vi "ER2007 Background DAQ Loop.vi"() -> ()   [LabVIEW 2013]
uses:
  <vilib>/Platform/TimedLoop/XDataNode/timing_clust.ctl
  <vilib>/Platform/TimedLoop/XDataNode/nitl_modes.ctl
  <vilib>/Platform/TimedLoop/XDataNode/wakeup.ctl
  <vilib>/DAQmx/read.llb/DAQmx Read (Analog 2D DBL NChan NSamp).vi
  <vilib>/Analysis/baseanly.llb/Mean (DBL).vi
  Controls/Global ER2007.vi
  <vilib>/DAQmx/create/channels.llb/DAQmx Create Channel (AI-Voltage-Basic).vi
  <vilib>/DAQmx/configure/timing.llb/DAQmx Timing (Sample Clock).vi
  <vilib>/DAQmx/miscellaneous.llb/DAQmx Fill In Error Info.vi
  <vilib>/platform/TimedLoop/XDataNode/XDataNode.xnode
  <vilib>/Analysis/NI_AALBase.lvlib
  <resource>/objmgr/daqmx.rc
  <vilib>/Platform/TimedLoop/XDataNode/XDNodeRunTimeDep.lvlib
panel:
  in  "T= Log Error":bool=TRUE
  in  "T=Notify":bool=TRUE
  in  "T=Notify":bool=TRUE
  in  "ThermocoupleType":u16(ring)=3 items=["B", "E", "J", "K", "R", "S", "T", "N"]
  out "Dev2 Err":bool
  out "Volts 2":dbl[](array[numeric]) format="%.4f"
  out "EUs 2":dbl[](array[numeric]) format="%.3f"
  out "NumCals 2":i32=28
  out "msec 3":u32=102
  in  "PhyChls 2":tag="Dev2/ai0:3, Dev2/ai5:11, Dev2/ai13:19, Dev2/ai21:27, Dev2/ai29:31"
  in  "MaxVolts 2":dbl=5.0 format="%0.2f"
  in  "MiinVolts 2":dbl=-5.0 format="%0.2f"
  in  "InputCfg 2":i32(ring)=10083 items=["default"=-1, "RSE"=10083, "NRSE"=10078, "Differential"=10106, "Pseudodifferential"=12529]
  in  "Rate 2":dbl=1000.0
  in  "SampleMode 2":i32(ring)=10178 items=["Finite Samples"=10178, "Continuous Samples"=10123, "Hardware Timed Single Point"=12522]
  in  "Samps/Chl 2":i32=100
  out "NumChls 3":i32=28
  out "ActRate 2":dbl format="%.2f"
  out "Sample 2":bool
  out "Galil Err":bool
  out "Dev1 Err":bool
  out "EUs 1":dbl[](array[numeric]) format="%.3f"
  out "Sample 1":bool
  out "Query":bool
  out "NumCtrls":i32
  in  "Controller #'s":u16[](array[numeric])=[1, 1, 1, 1, 1]
  out "msec 2":u32=102
  out "msec 1":u32=102
  out "ActRate":dbl format="%.2f"
  out "EUs 3":dbl[](array[numeric]) format="%.2f"
  in  "TC & CJ-1 Idxs":i32[][](array[numeric])=[[1, 5], [2, 6], [8, 15], [9, 16], [12, 19], [13, 20], [22, 29], [23, 30], [26, 33], [27, 34]]
  out "NumCals 3":i32=10
  out "NumCals 1":i32=7
  out "Late":bool
  out "Volts 1":dbl[](array[numeric]) format="%.4f"
  out "NumChls 3":i32=10
  out "NumChls 1":i32=7
  in  "Devs":T1(ring)=enum."All"
  in  "Period 3":dbl=60.0 caption="(secs)"
  out "ErrOut":errorcluster
  in  "Samps/Chl 1":i32=100
  in  "SampleMode 1":i32(ring)=10178 items=["Finite Samples"=10178, "Continuous Samples"=10123, "Hardware Timed Single Point"=12522]
  in  "Rate 1":dbl=1000.0
  in  "InputCfg 1":i32(ring)=10083 items=["default"=-1, "RSE"=10083, "NRSE"=10078, "Differential"=10106, "Pseudodifferential"=12529]
  in  "MiinVolts 1":dbl=-5.0 format="%0.2f"
  in  "MaxVolts 1":dbl=5.0 format="%0.2f"
  in  "SimOn":bool
  in  "Stop":bool
  in  "PhyChls 1":tag="Dev1/ai0:3, Dev1/ai8:10"
  in  "Init":bool
  # "Dev 1"
  # "Galil CDS-3310"
  # "Note: Max rate is about 8333 Hz (250 Khz / 30 chls)"
  # "Pvol1"
  # "Pdp2"
  # "Pvol2"
  # "Pdp3"
  # "Pdp4"
  # "Pdp5"
  # "Pvol5"
  # "Dev 2"
  # "Galil Assignments\n\nNet Chl  Chl Desc  Dev Out Idx  Both Dev Idx\n-------  --------  -----------  ------------\nNet 0.1   DelP1          0           35\nNet 0.2    Vol1          1           36\nNet 1.1   Delp2          2           37\nNet 1.2    Vol2          3           38\nNet 2.1   DelP3          4           39\nNet 2.2    Vol3          5           40\nNet 3.1   DelP4          6           41\nNet 3.2    Vol4          7           42\nNet 4.1   DelP5          8           43\nNet 4.2    Vol5          9           44"
  # "Old ER2006 Dev 1 Assignments\n\nA/D Chl  Chl Desc  Dev Out Idx  Both Dev Idx\n-------  --------  -----------  ------------\n    0      NOP1          0            0\n    1      TC1A          1            1\n    2      TC1B          2            2\n    3      NOP2          3            3\n    4      TC2A          4            4\n    5      TC2B          5            5\n    6      NOP3          6            6\n    7    <spare>         -            -\n    8       Pc1          7            7\n    9      CJ1A          8            8\n   10      CJ1B          9            9\n   11       Pc2         10           10\n   12      CJ2A         11           11\n   13      CJ2B         12           12\n   14       Pc3         13           13\n   15    <spare>         -            -\n   16      TC3A         14           14\n   17      TC3B         15           15\n   18      NOP4         16           16\n   19      TC4A         17           17\n   20      TC4B         18           18\n   21      NOP5         19           19\n   22      TC5A         20           20\n   23      TC5B         21           21\n   24      CJ3A         22           22\n   25      CJ3B         23           23\n   26       Pc4         24           24\n   27      CJ4A         25           25\n   28      CJ4B         26           26\n   29       Pc5         27           27\n   30      CJ5A         28           28\n   31      CJ5B         29           29"
  # "Dev 1 PCI-6220 Assignments\n\nA/D Chl  Chl Desc  Dev Out Idx  Both Dev Idx\n-------  --------  -----------  ------------\n    0      NOP1          0            0\n    1      TC1A          1            1\n    2      TC1B          2            2\n    3      Pc1B          3            3\n    4    <spare>         -            -\n    5    <spare>         -            -\n    6    <spare>         -            -\n    7    <spare>         -            -\n    8      Pc1A          4            4\n    9      CJ1A          5            5\n   10      CJ1B          6            6"
  # "Dev 2 PCI-6224 Assignments\n\nA/D Chl  Chl Desc  Dev Out Idx  Both Dev Idx\n-------  --------  -----------  ------------\n    0      NOP2          0            7\n    1      TC2A          1            8\n    2      TC2B          2            9\n    3      Pc2B          3           10\n    4    <spare>         -            -\n    5      Pc3A          4           11\n    6      TC3A          5           12\n    7      TC3B          6           13\n    8      Pc2A          7           14\n    9      CJ2A          8           15\n   10      CJ2B          9           16\n   11      NOP3         10           17\n   12    <spare>         -            -\n   13      Pc3B         11           18\n   14      CJ3A         12           19\n   15      CJ3B         13           20\n   16      NOP4         14           21\n   17      TC4A         15           22\n   18      TC4B         16           23\n   19      Pc4B         17           24\n   20    <spare>         -            -\n   21      Pc5A         18           25\n   22      TC5A         19           26\n   23      TC5B         20           27\n   24      Pc4A         21           28\n   25      CJ4A         22           29\n   26      CJ4B         23           30\n   27      NOP5         24           31\n   28    <spare>         -            -\n   29      Pc5B         25           32\n   30      CJ5A         26           33\n   31      CJ5B         27           34"
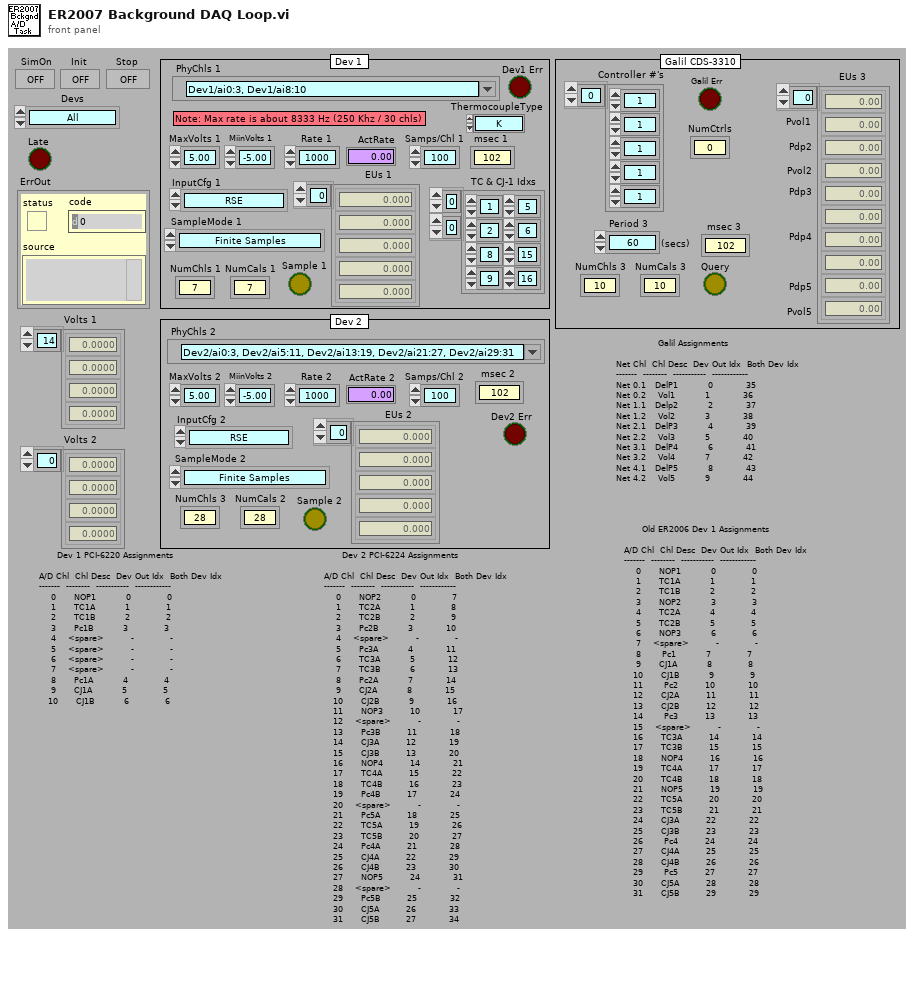
[diagram p1: front panel]
types:
  T1 = enum16{"Dev 1", "Dev 2", "Dev 1 & Dev 2", "Galil", "All"}
  T2 = typedef "XDNodeRunTimeDep.lvlib/timing_clust.ctl" = cluster{"Expected End [f-1]":u64, "Actual End [f-1]":u64, "Finished Late? [f-1]":bool, "Expected End [i-1]":u64, "Actual End [i-1]":u64, "Finished Late? [i-1]":bool, "Expected Start [i]":u64, "Actual Start [i]":u64, "Expected Start [f]":u64, "Actual Start [f]":u64, "Source Name":string, "Structure Name":string, "Period":i64, "Deadline":i64, "Offset":i64, "Start":i64, "Priority":i32, "Timeout":i32, "Mode":T3, "Wakeup Reason":T4, "Error":errorcluster, "Source Type":string, "Secondary Source Type":string, "Global End Time":u64, "Global Start Time":u64, "Frame Duration":u64, "Iteration Duration":u64, "Assigned CPU":i32, "I/O Scan Engine Mode":u32}
  T3 = typedef "XDNodeRunTimeDep.lvlib/nitl_modes.ctl" = enum32{"No Change", "Process missed periods, maintain original phase", "Discard missed periods, maintain original phase", "Process missed periods, ignore original phase", "Discard missed periods, ignore original phase"}
  T4 = typedef "XDNodeRunTimeDep.lvlib/wakeup.ctl" = enum32{"Normal", "Aborted", "Asynchronous wakeup", "Timing source error", "Timed loop error", "Timeout"}
  T5 = cluster{"PageTitle":string, "NumLines":i32, "ChlNum":string[], "ChlDesc":string[], "ChlUnits":string[], "ChlZero":sgl[], "ChlFactor":sgl[], "ChlConfig":u16[]}[]
  T6 = cluster{"PageTitle":string, "NumLines":i32, "ChlNum":string[], "ChlDesc":string[], "ChlUnits":string[], "ChlZero":sgl[], "ChlFactor":sgl[], "ChlConfig":u16[]}
  T7 = enum16{"Cell 1", "Cell 2", "Cell 3", "Cell 4", "Cell 5"}
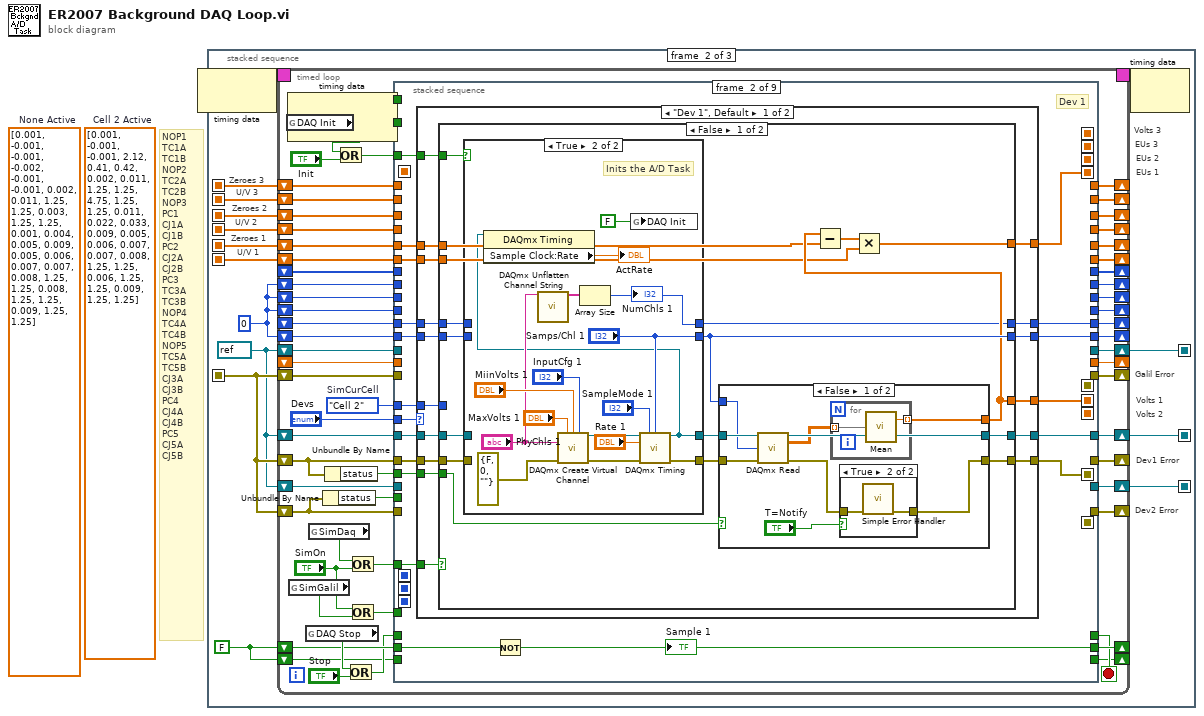
[diagram p0: block diagram]
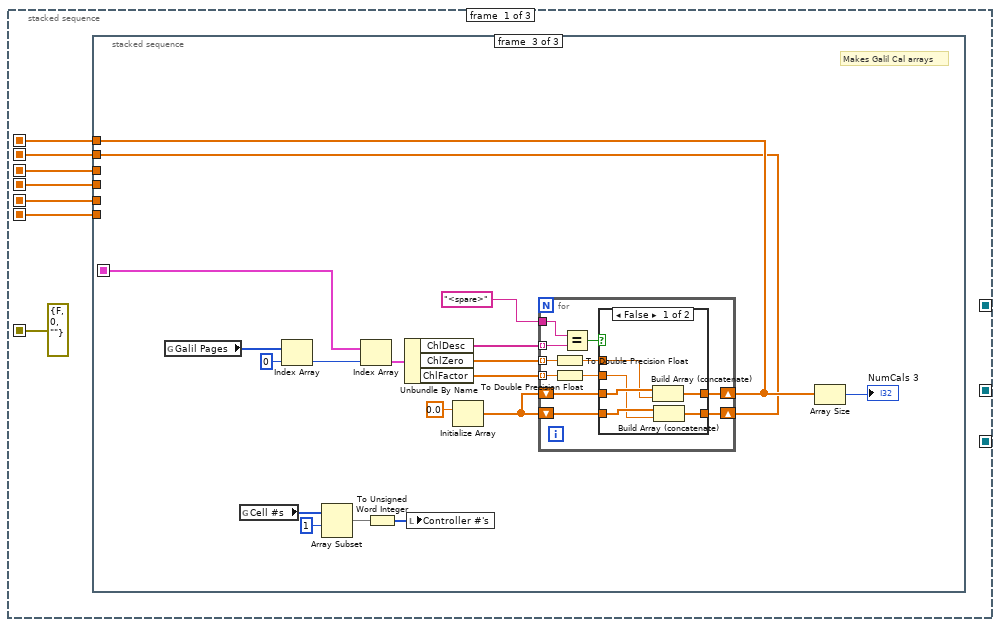
[diagram p2: hidden frame]
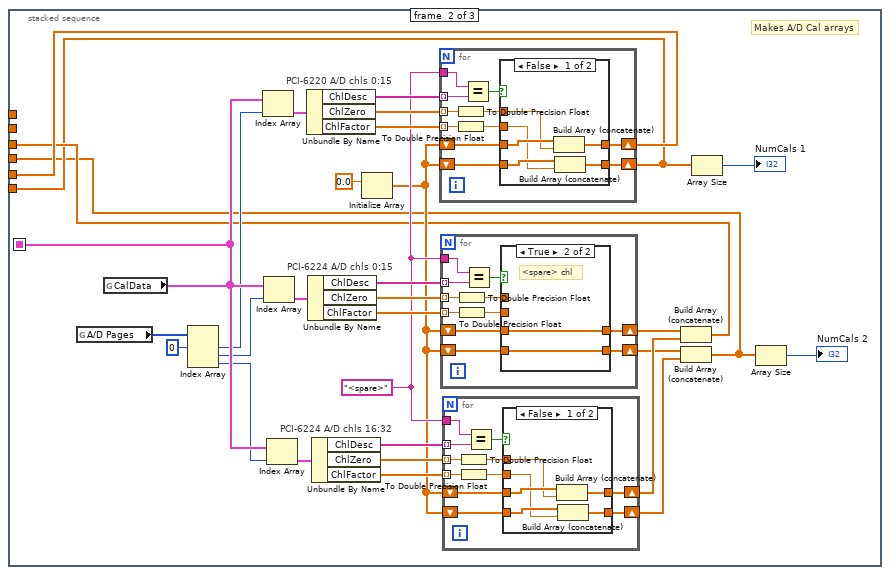
[diagram p4: hidden frame]
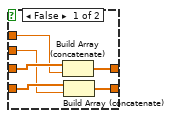
[diagram p7: hidden frame]
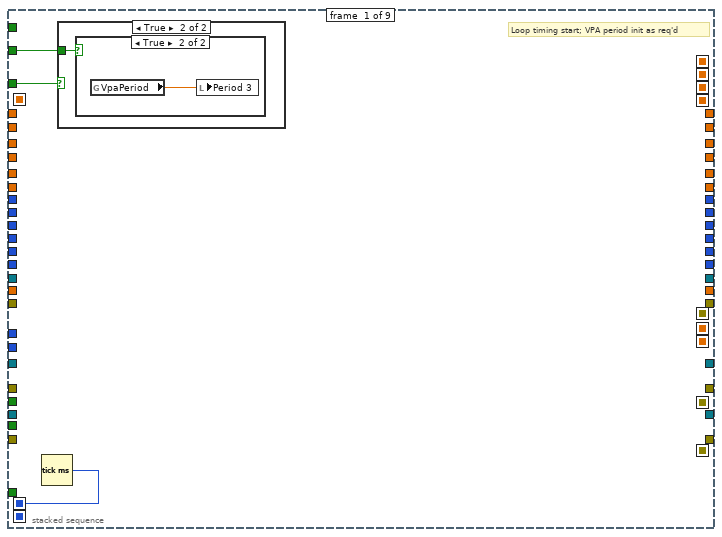
[diagram p9: hidden frame]
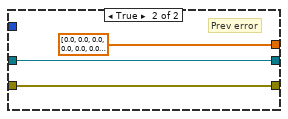
[diagram p13: hidden frame]
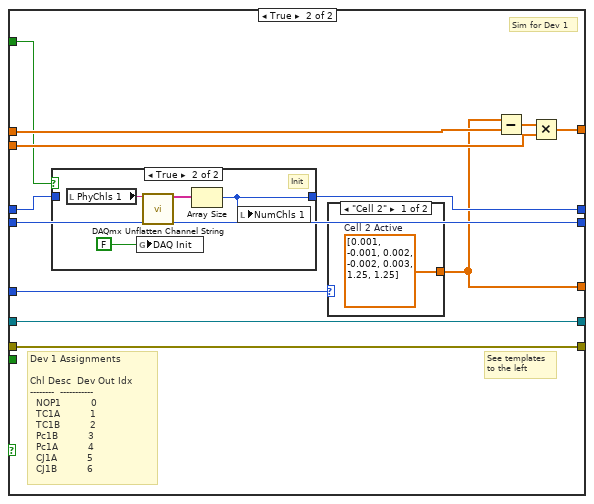
[diagram p15: hidden frame]
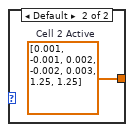
[diagram p16: hidden frame]
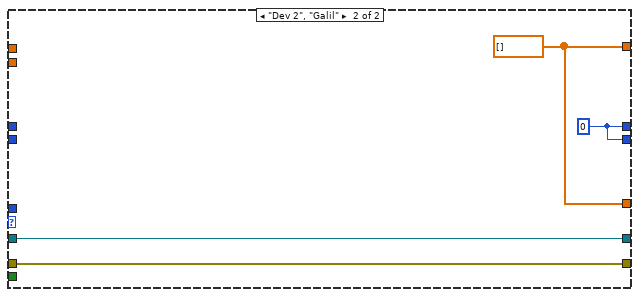
[diagram p18: hidden frame]
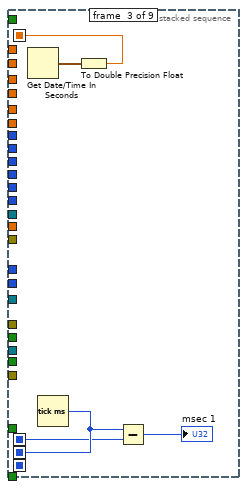
[diagram p19: hidden frame]
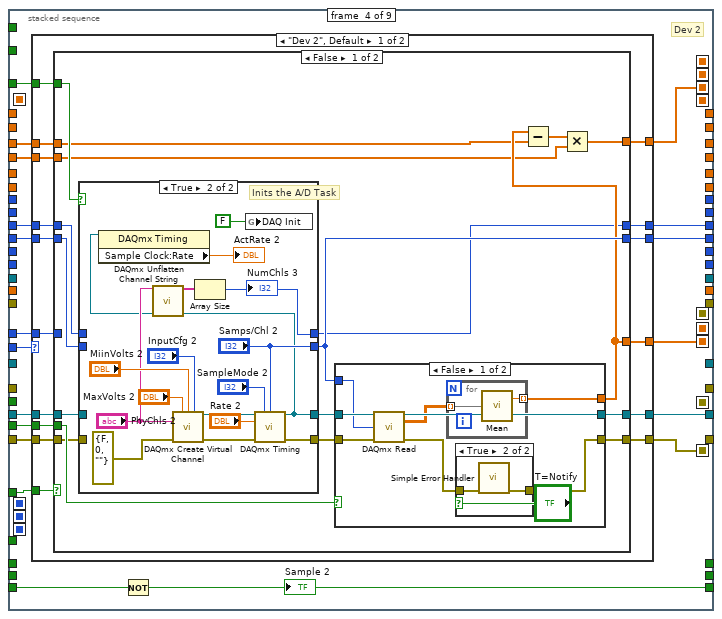
[diagram p20: hidden frame]
diagram:
  (unwired) dbl[] [0.001, -0.001, -0.001, 2.12, 0.41, 0.42, 0.002, 0.011, 1.25, 1.25, 4.75, 1.25, 1.25, 0.011, 0.022, 0.033, 0.009, 0.005, 0.006, 0.007, 0.007, 0.008, 1.25, 1.25, 0.006, 1.25, 1.25, 0.009, 1.25, 1.25]  # Cell 2 Active
  (unwired) dbl[] [0.001, -0.001, -0.001, -0.002, -0.001, -0.001, 0.002, 0.011, 1.25, 1.25, 0.003, 1.25, 1.25, 0.001, 0.004, 0.005, 0.009, 0.005, 0.006, 0.007, 0.007, 0.008, 1.25, 1.25, 0.008, 1.25, 1.25, 0.009, 1.25, 1.25]  # None Active
  # "NOP1\nTC1A\nTC1B\nNOP2\nTC2A\nTC2B\nNOP3\nPC1\nCJ1A\nCJ1B\nPC2\nCJ2A\nCJ2B\nPC3\nTC3A\nTC3B\nNOP4\nTC4A\nTC4B\nNOP5\nTC5A\nTC5B\nCJ3A\nCJ3B\nPC4\nCJ4A\nCJ4B\nPC5\nCJ5A\nCJ5B"
  n1 = stacked-sequence {
    seq-local: [w3 _ _] -> [_ w136 _]
    seq-local: [w7 _ _] -> [_ w135 _]
    seq-local: [_ w147 _] -> [_ _ w876]
    seq-local: [w5 _ _] -> [_ w140 _]
    seq-local: [w6 _ _] -> [_ w139 _]
    seq-local: [_ w146 _] -> [_ _ w875]
    seq-local: [errorcluster {"status"=FALSE, "code"=0, "source"=""} ("error out") _ _] -> [_ w145 _]
    seq-local: [w2 _ _] -> [_ w138 _]
    seq-local: [w1 _ _] -> [_ w137 _]
    seq-local: [_ w141 _] -> [_ _ w873]
    frame #0 {
      n2 = stacked-sequence {
        seq-local: [_ w19 _] -> [_ _ w100]
        tunnel: [_ w11 _] -> w3
        tunnel: [_ w9 _] -> w7
        tunnel: [_ _ w98] -> w6
        tunnel: [_ _ w99] -> w5
        tunnel: [_ w10 _] -> w2
        tunnel: [_ w8 _] -> w1
        frame #0 {
          # "Notes and such"
          # "ERROR HANDLING\n\nTwo types of errors are reported: A/D errors and Galil (VPA) errors.  Each of the two\ncode sections has its own error cluster which are are checked in frame #5.  Errors are\nreported to the Main Test Panel using two separate globals.\n\nA/D Errors\n----------\nA/D errors do not generally occur once the code is optimized and tested for the first time.\nErrors that do occur after initial testing are generally fatal and hardware related.  There\nis no attempt inside the A/D code to correct for errors or write errors to the error log file.\nA/D sample rates are about 1000 samples per seconds.\n\nOnce an A/D error occurs, the error is latched until the problem is fixed and either the\n\"Reset DAQ\" is pressed on the Main Test Panel or the program is restarted.\n\nGalil Errors\n------------\nGalil errors are much more common and arise from communication errors due to collisions or\ntimeouts, and to the user tinkering with the VPA hardware or software configuration.  Not only\nare genuine errors possible but the user can change the data collection method from auto-VPA\npolling to Manual on any of the five VPA's on-the-fly.  This Auto/Manual switch is handled\ninternally in the five VPA vi's.  VPA polling occurs at 60 second intervals.\n\nAfter an error occurs it is latched until a subsequent poll is successfully completed at which\ntime the error is automatically cleared.  During polling, the first VPA to report an error is\nlatched; polling of higher numbered VPA's continues as though there were no error in an effort\nto collect data from working VPA's.  Errors in higher numbered VPA's are not reported if an\nerror occurred in a lower numbered one.\n\nError Logging\n-------------\nLogging errors to an error file is done only for VPA errors.  Only the first error of\nsuccessive errors is logged; a \"no-error\" poll resets the error logging vi and re-arms it."
        }
        frame #1 {
          w18 = "<spare>" ("x")
          # "PCI-6220 A/D chls 0:15"
          # "Makes A/D Cal arrays"
          # "PCI-6224 A/D chls 16:32"
          # "PCI-6224 A/D chls 0:15"
          n3 = global read "Global ER2007.vi" "A/D Pages"() -> (w28:i32[])
          n4 = global read "Global ER2007.vi" "CalData"() -> (w19:T5)
          n5 = Index Array(array=w28, index #1=0 ("index")) -> (element #1=w14:i32, element #2=w15:i32, element #3=w16:i32)  [unwired: 2 in]
          n6 = Index Array(array=w19, index=w14) -> (element=w23:T6)
          n7 = Index Array(array=w19, index=w15) -> (element=w36:T6)
          n8 = Index Array(array=w19, index=w16) -> (element=w38:T6)
          n9 = Unbundle By Name(w23) -> ("ChlDesc"=w22:string[], "ChlZero"=w21:sgl[], "ChlFactor"=w20:sgl[])
          n10 = Unbundle By Name(w36) -> ("ChlDesc"=w35:string[], "ChlZero"=w34:sgl[], "ChlFactor"=w33:sgl[])
          n11 = Unbundle By Name(w38) -> ("ChlDesc"=w29:string[], "ChlZero"=w30:sgl[], "ChlFactor"=w31:sgl[])
          n12 = Initialize Array(0.0 ("element")) -> (w17:dbl[])  [unwired: 1 in]
          n13 = for {
            tunnel: w22 -> [w49] mode=indexing
            tunnel: w21 -> [w42] mode=indexing
            tunnel: w20 -> [w41] mode=indexing
            tunnel: w18 -> [w48]
            shift-right: [w45] -> w11
            shift-left: w17 -> [w46]
            shift-right: [w43] -> w9
            shift-left: w17 -> [w44]
            n14 = To Double Precision Float(number=w42) -> (double precision float=w40:dbl)
            n15 = To Double Precision Float(number=w41) -> (double precision float=w39:dbl)
            n16 = Equal?(x=w48, y=w49) -> (x = y?=w47:bool)
            n17 = case shown="False" w47 {
              tunnel: w46 -> [w55 w57]
              tunnel: [w53 w57] -> w45
              tunnel: w44 -> [w51 w56]
              tunnel: [w52 w56] -> w43
              tunnel: w40 -> [w54 _]
              tunnel: w39 -> [w50 _]
              frame False {
                n18 = Build Array (concatenate)(w55, w54) -> (w53:dbl[])
                n19 = Build Array (concatenate)(w51, w50) -> (w52:dbl[])
              }
              frame True {
                # "<spare> chl"
              }
            }
          }
          n20 = for {
            tunnel: w35 -> [w87] mode=indexing
            tunnel: w34 -> [w80] mode=indexing
            tunnel: w33 -> [w79] mode=indexing
            tunnel: w18 -> [w86]
            shift-right: [w83] -> w26
            shift-left: w17 -> [w84]
            shift-right: [w81] -> w24
            shift-left: w17 -> [w82]
            n21 = To Double Precision Float(number=w80) -> (double precision float=w78:dbl)
            n22 = To Double Precision Float(number=w79) -> (double precision float=w77:dbl)
            n23 = Equal?(x=w86, y=w87) -> (x = y?=w85:bool)
            n24 = case shown="True" w85 {
              tunnel: w84 -> [w93 w95]
              tunnel: [w91 w95] -> w83
              tunnel: w82 -> [w89 w94]
              tunnel: [w90 w94] -> w81
              tunnel: w78 -> [w92 _]
              tunnel: w77 -> [w88 _]
              frame False {
                n25 = Build Array (concatenate)(w93, w92) -> (w91:dbl[])
                n26 = Build Array (concatenate)(w89, w88) -> (w90:dbl[])
              }
              frame True {
                # "<spare> chl"
              }
            }
          }
          n27 = for {
            tunnel: w29 -> [w68] mode=indexing
            tunnel: w30 -> [w61] mode=indexing
            tunnel: w31 -> [w60] mode=indexing
            tunnel: w18 -> [w67]
            shift-right: [w64] -> w27
            shift-left: w17 -> [w65]
            shift-right: [w62] -> w25
            shift-left: w17 -> [w63]
            n28 = To Double Precision Float(number=w61) -> (double precision float=w59:dbl)
            n29 = To Double Precision Float(number=w60) -> (double precision float=w58:dbl)
            n30 = Equal?(x=w67, y=w68) -> (x = y?=w66:bool)
            n31 = case shown="False" w66 {
              tunnel: w65 -> [w74 w76]
              tunnel: [w72 w76] -> w64
              tunnel: w63 -> [w70 w75]
              tunnel: [w71 w75] -> w62
              tunnel: w59 -> [w73 _]
              tunnel: w58 -> [w69 _]
              frame False {
                n32 = Build Array (concatenate)(w74, w73) -> (w72:dbl[])
                n33 = Build Array (concatenate)(w70, w69) -> (w71:dbl[])
              }
              frame True {
                # "<spare> chl"
              }
            }
          }
          n34 = Build Array (concatenate)(w26, w27) -> (w10:dbl[])
          n35 = Build Array (concatenate)(w24, w25) -> (w8:dbl[])
          n36 = Array Size(array=w9) -> (size(s)=→"NumCals 1":i32)
          n37 = Array Size(array=w8) -> (size(s)=→"NumCals 2":i32)
        }
        frame #2 {
          # "Makes Galil Cal arrays"
          n38 = global read "Global ER2007.vi" "Galil Pages"() -> (w109:i32[])
          n39 = global read "Global ER2007.vi" "Cell #s"() -> (w105:i32[])
          n40 = Index Array(array=w109, index=0) -> (element=w107:i32)
          n41 = Array Subset(array=w105, index=1) -> (w103:i32[])  [unwired: 1 in]
          n42 = Index Array(array=w100, index=w107) -> (element=w113:T6)
          n43 = To Unsigned Word Integer(number=w103) -> (unsigned 16bit integer=w102:u16[])
          n44 = Unbundle By Name(w113) -> ("ChlDesc"=w112:string[], "ChlZero"=w111:sgl[], "ChlFactor"=w110:sgl[])
          n45 = local write "Controller #'s"(w102) -> ()
          n46 = Initialize Array(0.0 ("element")) -> (w96:dbl[])  [unwired: 1 in]
          n47 = for {
            tunnel: w112 -> [w124] mode=indexing
            tunnel: w111 -> [w117] mode=indexing
            tunnel: w110 -> [w116] mode=indexing
            tunnel: "<spare>" ("x") -> [w123]
            shift-right: [w120] -> w99
            shift-left: w96 -> [w121]
            shift-right: [w118] -> w98
            shift-left: w96 -> [w119]
            n48 = To Double Precision Float(number=w117) -> (double precision float=w115:dbl)
            n49 = To Double Precision Float(number=w116) -> (double precision float=w114:dbl)
            n50 = Equal?(x=w123, y=w124) -> (x = y?=w122:bool)
            n51 = case shown="False" w122 {
              tunnel: w121 -> [w130 w132]
              tunnel: [w128 w132] -> w120
              tunnel: w119 -> [w126 w131]
              tunnel: [w127 w131] -> w118
              tunnel: w115 -> [w129 _]
              tunnel: w114 -> [w125 _]
              frame False {
                n52 = Build Array (concatenate)(w130, w129) -> (w128:dbl[])
                n53 = Build Array (concatenate)(w126, w125) -> (w127:dbl[])
              }
              frame True {
                # "<spare> chl"
              }
            }
          }
          n54 = Array Size(array=w99) -> (size(s)=→"NumCals 3":i32)
        }
      }
    }
    frame #1 {
      w143 = FALSE ("Sample")
      w142 = 0 ("Samps/Chl")
      w144 = refnum<k21> refnum ("task out")
      # "Dev2 Error"
      # "Dev1 Error"
      # "Galil Error"
      # "Volts 3"
      # "EUs 3"
      # "Volts 2"
      # "EUs 2"
      # "Volts 1"
      # "EUs 1"
      # "U/V 2"
      # "Zeroes 2"
      # "U/V 3"
      # "Zeroes 3"
      # "Zeroes 1"
      # "U/V 1"
      n55 = node-c288() -> (w133:T2)  [unwired: 1 in]
      n56 = timed-loop {
        shift-left: w135 -> [w153]
        shift-right: [w152] -> _
        shift-left: w136 -> [w154]
        shift-right: [w149] -> _
        shift-left: w137 -> [w156]
        shift-right: [w155] -> _
        shift-left: w138 -> [w157]
        shift-right: [w150] -> _
        shift-left: w139 -> [w159]
        shift-right: [w151] -> _
        shift-left: w140 -> [w160]
        shift-right: [w158] -> _
        shift-left: w142 -> [w165]
        shift-right: [w163] -> _
        shift-left: w142 -> [w164]
        shift-right: [w162] -> _
        shift-left: w143 -> [w171]
        shift-right: [w170] -> _
        shift-left: w145 -> [w169]
        shift-right: [w161] -> _
        shift-left: w144 -> [w173]
        shift-right: [w172] -> w141
        shift-left: w143 -> [w177]
        shift-right: [w178] -> _
        shift-left: _ -> [w180]
        shift-right: [w179] -> _
        shift-left: _ -> [w190]
        shift-right: [w191] -> _
        shift-left: _ -> [w192]
        shift-right: [w193] -> _
        shift-left: w144 -> [w197]
        shift-right: [w196] -> w146
        shift-left: w145 -> [w188]
        shift-right: [w198] -> _
        shift-left: w142 -> [w200]
        shift-right: [w199] -> _
        shift-left: w142 -> [w195]
        shift-right: [w202] -> _
        shift-left: w144 -> [w166]
        shift-right: [w203] -> w147
        shift-left: w145 -> [w168]
        shift-right: [w174] -> _
        timing-out: [_] -> w134
        timing: w133 -> [_]
        stop <- w175 stop-if-true
        w186 = T7."Cell 2"  # SimCurCell
        n57 = global read "Global ER2007.vi" "DAQ Init"() -> (w148:bool)
        n58 = node-c288() -> (w189:bool)  [unwired: 1 in, 1 out]
        n59 = global read "Global ER2007.vi" "SimGalil"() -> (w183:bool)
        n60 = global read "Global ER2007.vi" "DAQ Stop"() -> (w184:bool)
        n61 = global read "Global ER2007.vi" "SimDaq"() -> (w185:bool)
        n62 = Unbundle By Name(w169) -> ("status"=w187:bool)
        n63 = Unbundle By Name(w168) -> ("status"=w167:bool)
        n64 = Or(x=w148, y="Init") -> (x .or. y?=w205:bool)
        n65 = Or(x=w184, y="Stop") -> (x .or. y?=w176:bool)
        n66 = Or(x=w185, y="SimOn") -> (x .or. y?=w201:bool)
        n67 = Or(x="SimOn", y=w183) -> (x .or. y?=w181:bool)
        n68 = stacked-sequence {
          seq-local: [_ w226 _ _ _ _ _ _ _] -> [_ _ _ _ _ _ _ w685 _]
          seq-local: [_ w225 _ _ _ _ _ _ _] -> [_ _ _ _ _ _ _ w703 _]
          seq-local: [_ _ _ _ _ w451 _ _ _] -> [_ _ _ _ _ _ _ w684 _]
          seq-local: [w211 _ _ _ _ _ _ _ _] -> [_ _ w329 _ _ _ _ _ _]
          seq-local: [_ _ w330 _ _ _ _ _ _] -> [_ _ _ _ w445 _ _ _ _]
          seq-local: [_ _ _ _ _ w450 _ _ _] -> [_ _ _ _ _ _ _ w688 _]
          seq-local: [_ _ w326 _ _ _ _ _ _] -> [_ _ _ _ _ w448 _ _ _]
          seq-local: [_ w216 _ _ _ _ _ _ _] -> [_ _ _ _ _ _ _ w683 _]
          seq-local: [_ _ _ _ _ w446 _ _ _] -> [_ _ _ _ _ _ _ w691 _]
          seq-local: [_ _ _ w343 _ _ _ _ _] -> [_ _ _ _ _ _ _ w682 _]
          seq-local: [_ _ _ _ w444 _ _ _ _] -> [_ _ _ _ _ _ w674 _ _]
          seq-local: [_ _ _ w334 _ _ _ _ _] -> [_ _ _ _ _ _ _ w687 _]
          seq-local: [_ _ _ w331 _ _ _ _ _] -> [_ _ _ _ _ _ _ w678 _]
          tunnel: w205 -> [w210 w232 _ w349 _ w465 _ _ _]
          tunnel: [_ w224 _ _ _ _ _ _ _] -> w203
          tunnel: w168 -> [_ w231 _ _ _ _ _ _ _]
          tunnel: [_ w230 _ _ _ _ _ _ _] -> w202
          tunnel: w201 -> [_ w229 _ w348 _ _ _ _ _]
          tunnel: w173 -> [_ _ _ w347 _ _ _ _ _]
          tunnel: w200 -> [_ _ _ _ _ w464 _ _ _]
          tunnel: w154 -> [_ w228 _ _ _ _ _ _ w731]
          tunnel: w153 -> [_ w227 _ _ _ _ _ _ w730]
          tunnel: w160 -> [_ _ _ _ _ w463 _ _ w737]
          tunnel: w159 -> [_ _ _ _ _ w462 _ _ w736]
          tunnel: [_ _ _ _ _ w461 _ _ _] -> w199
          tunnel: w188 -> [_ _ _ _ _ w460 _ _ _]
          tunnel: [_ _ _ _ _ _ _ w690 _] -> w198
          tunnel: w197 -> [_ _ _ _ _ w459 _ _ _]
          tunnel: [_ _ _ _ _ w458 _ _ _] -> w196
          tunnel: w195 -> [_ w223 _ _ _ _ _ _ _]
          tunnel: "Devs" -> [_ w222 _ w346 _ w457 _ _ _]
          tunnel: [_ w221 _ _ _ _ _ _ _] -> w193
          tunnel: w192 -> [_ w220 _ _ _ _ _ _ _]
          tunnel: [_ _ _ _ _ w456 _ _ _] -> w191
          tunnel: w190 -> [_ _ _ _ _ w455 _ _ _]
          tunnel: w189 -> [_ _ _ _ _ _ _ w702 _]
          tunnel: w187 -> [_ _ _ w345 _ _ _ _ _]
          tunnel: w186 -> [_ w219 _ w344 _ w454 _ _ _]
          tunnel: w181 -> [_ _ _ _ _ w453 _ _ _]
          tunnel: w180 -> [_ _ _ _ _ w452 _ _ _]
          tunnel: [_ _ _ _ _ w449 _ _ _] -> w179
          tunnel: [_ w217 _ _ _ _ _ _ _] -> w178
          tunnel: w177 -> [_ w218 _ _ _ _ _ _ _]
          tunnel: w176 -> [_ _ _ _ _ w447 _ w693 _]
          tunnel: [_ _ _ _ _ _ _ w693 _] -> w175
          tunnel: [_ _ _ _ _ _ _ w683 _] -> w174
          tunnel: [_ _ _ w342 _ _ _ _ _] -> w172
          tunnel: w171 -> [_ _ _ w341 _ _ _ _ _]
          tunnel: [_ _ _ w340 _ _ _ _ _] -> w170
          tunnel: w169 -> [_ _ _ w339 _ _ _ _ _]
          tunnel: w167 -> [_ w215 _ _ _ _ _ _ _]
          tunnel: w166 -> [_ w214 _ _ _ _ _ _ _]
          tunnel: w165 -> [_ _ _ w338 _ _ _ _ _]
          tunnel: w164 -> [_ _ _ w337 _ _ _ _ _]
          tunnel: [_ _ _ w336 _ _ _ _ _] -> w163
          tunnel: [_ _ _ w335 _ _ _ _ _] -> w162
          tunnel: w157 -> [_ _ _ w333 _ _ _ _ w734]
          tunnel: w156 -> [_ _ _ w332 _ _ _ _ w733]
          tunnel: [_ _ _ _ _ _ _ w682 _] -> w161
          tunnel: [_ _ _ _ _ _ _ _ w735] -> w158
          tunnel: [_ _ _ _ _ _ _ _ w732] -> w155
          tunnel: [_ _ _ _ _ _ _ _ w729] -> w152
          tunnel: [_ _ _ _ _ _ _ _ w728] -> w151
          tunnel: [_ _ _ _ _ _ _ _ w727] -> w150
          tunnel: [_ _ _ _ _ _ _ _ w726] -> w149
          tunnel: w148 -> [w209 _ _ _ _ _ _ _ _]
          frame #0 {
            # "Loop timing start; VPA period init as req'd"
            n69 = Tick Count (ms)() -> (millisecond timer value=w211:u32)
            n70 = case shown="True" w210 {
              tunnel: w209 -> [_ w212]
              frame False {
              }
              frame True {
                n71 = case shown="True" w212 {
                  frame False {
                  }
                  frame True {
                    n72 = global read "Global ER2007.vi" "VpaPeriod"() -> (w213:dbl)
                    n73 = local write "Period 3"(w213) -> ()
                  }
                }
              }
            }
          }
          frame #1 {
            # "Dev 1"
            n74 = case shown="\"Dev 1\", Default" w222 {
              tunnel: w232 -> [w248 _]
              tunnel: w231 -> [w247 w323]
              tunnel: [w246 w322] -> w230
              tunnel: w229 -> [w245 _]
              tunnel: w214 -> [w244 w324]
              tunnel: w228 -> [w243 _]
              tunnel: w227 -> [w242 _]
              tunnel: w215 -> [w241 _]
              tunnel: [w240 w325] -> w226
              tunnel: [w239 w325] -> w225
              tunnel: [w238 w324] -> w224
              tunnel: [w237 w323] -> w216
              tunnel: w223 -> [w236 _]
              tunnel: [w235 w322] -> w221
              tunnel: w220 -> [w234 _]
              tunnel: w219 -> [w233 _]
              frame "Dev 1", Default {
                n75 = case shown="False" w245 {
                  tunnel: w248 -> [w265 w306]
                  tunnel: [w263 w314] -> w237
                  tunnel: [w261 w313] -> w238
                  tunnel: w247 -> [w260 w314]
                  tunnel: w241 -> [w259 _]
                  tunnel: [w258 w312] -> w246
                  tunnel: [w257 w304] -> w239
                  tunnel: w244 -> [w251 w313]
                  tunnel: w236 -> [w252 w312]
                  tunnel: [w253 w310] -> w240
                  tunnel: w243 -> [w256 w309]
                  tunnel: w242 -> [w254 w308]
                  tunnel: [w250 w305] -> w235
                  tunnel: w234 -> [w249 w307]
                  tunnel: w233 -> [_ w303]
                  frame False {
                    n76 = case shown="True" w265 {
                      tunnel: w260 -> [w284 _]
                      tunnel: [w284 w300] -> w264
                      tunnel: [w285 w290] -> w262
                      tunnel: [w286 "Samps/Chl 1"] -> w258
                      tunnel: w252 -> [w286 _]
                      tunnel: w251 -> [w285 _]
                      tunnel: [w283 w291] -> w250
                      tunnel: w249 -> [w283 _]
                      frame False {
                      }
                      frame True {
                        # "Inits the A/D Task"
                        n77 = call <vilib>:"DAQmx Unflatten Channel String.vi"("names in"="PhyChls 1") -> ("names out"=w292:string[])  [unwired: 13 in, 1 out]
                        n78 = call-poly <vilib>:"DAQmx Create Virtual Channel.vi"("maximum value"="MaxVolts 1", "minimum value"="MiinVolts 1", "input terminal configuration"="InputCfg 1", "physical channels"="PhyChls 1", "error in"=errorcluster {"status"=FALSE, "code"=0, "source"=""}) -> ("task out"=w301:refnum<k21>, "error out"=w302:errorcluster)  [unwired: 9 in]
                        n79 = Array Size(array=w292) -> (size(s)=w291:i32)
                        "NumChls 1" <- w291
                        n80 = global write "Global ER2007.vi" "DAQ Init"(FALSE ("A/D Init")) -> ()
                        n81 = call-poly <vilib>:"DAQmx Timing.vi"("task/channels in"=w301, "sample mode"="SampleMode 1", "samples per channel"="Samps/Chl 1", "rate"="Rate 1", "error in"=w302) -> ("task out"=w290:refnum<k21>, "error out"=w300:errorcluster)  [unwired: 9 in]
                        n82 = property class="DAQmx Timing"(reference=w290) -> ("Sample Clock:Rate"=→"ActRate":dbl)  [unwired: 1 in, 2 out]
                      }
                    }
                    n83 = case shown="False" w259 {
                      tunnel: w264 -> [w274 w281]
                      tunnel: w262 -> [w273 w282]
                      tunnel: [w272 w282] -> w261
                      tunnel: [w270 w281] -> w263
                      tunnel: [w269 dbl[] [0.0, 0.0, 0.0, 0.0, 0.0, 0.0, 0.0, 0.0, 0.0, 0.0, 0.0, 0.0] ("data")] -> w257
                      tunnel: w258 -> [w267 _]
                      frame False {
                        n84 = call-poly <vilib>:"DAQmx Read.vi"("task/channels in"=w273, "number of samples per channel"=w267, "error in"=w274) -> ("task out"=w272:refnum<k21>, "data"=w268:dbl[][], "error out"=w271:errorcluster)  [unwired: 10 in]
                        n85 = for {
                          tunnel: [w279] -> w269 mode=indexing
                          tunnel: w268 -> [w278] mode=indexing
                          n86 = call-poly <vilib>:"Mean.vi"("X"=w278) -> ("mean"=w279:dbl)  [unwired: 1 out]
                        }
                        n87 = case shown="True" "T=Notify" {
                          tunnel: w271 -> [w275 w277]
                          tunnel: [w275 w276] -> w270
                          frame False {
                          }
                          frame True {
                            n88 = call <vilib>:"Simple Error Handler.vi"("error in (no error)"=w277) -> ("error out"=w276:errorcluster)  [unwired: 4 in, 4 out]
                          }
                        }
                      }
                      frame True {
                        # "Prev error"
                      }
                    }
                    n89 = Subtract(x=w257, y=w256) -> (x-y=w255:dbl[])
                    n90 = Multiply(x=w255, y=w254) -> (x*y=w253:dbl[])
                  }
                  frame True {
                    # "See templates\nto the left"
                    # "Dev 1 Assignments\n\nChl Desc  Dev Out Idx\n--------  -----------\n  NOP1          0\n  TC1A          1\n  TC1B          2\n  Pc1B          3\n  Pc1A          4\n  CJ1A          5\n  CJ1B          6"
                    # "Sim for Dev 1"
                    n91 = case shown="True" w306 {
                      tunnel: w307 -> [w317 _]
                      tunnel: [w317 w319] -> w305
                      frame False {
                      }
                      frame True {
                        # "Init"
                        n92 = local read "PhyChls 1"() -> (w321:tag)
                        n93 = global write "Global ER2007.vi" "DAQ Init"(FALSE ("A/D Init")) -> ()
                        n94 = call <vilib>:"DAQmx Unflatten Channel String.vi"("names in"=w321) -> ("names out"=w320:string[])  [unwired: 13 in, 1 out]
                        n95 = Array Size(array=w320) -> (size(s)=w319:i32)
                        n96 = local write "NumChls 1"(w319) -> ()
                      }
                    }
                    n97 = case shown="\"Cell 2\"" w303 {
                      tunnel: [w315 w316] -> w304
                      frame "Cell 2" {
                        w315 = dbl[] [0.001, -0.001, 0.002, -0.002, 0.003, 1.25, 1.25]  # Cell 2 Active
                      }
                      frame Default {
                        w316 = dbl[] [0.001, -0.001, 0.002, -0.002, 0.003, 1.25, 1.25]  # Cell 2 Active
                      }
                    }
                    n98 = Subtract(x=w304, y=w309) -> (x-y=w311:dbl[])
                    n99 = Multiply(x=w311, y=w308) -> (x*y=w310:dbl[])
                  }
                }
              }
              frame "Dev 2", "Galil" {
                w325 = dbl[] []
                w322 = 0 ("Samps/Chl")
              }
            }
            n100 = Not(x=w218) -> (.not. x?=w217:bool)
            "Sample 1" <- w217
          }
          frame #2 {
            n101 = Get Date/Time In Seconds() -> (seconds since 1Jan1904=w327:timestamp)
            n102 = Tick Count (ms)() -> (millisecond timer value=w330:u32)
            n103 = To Double Precision Float(number=w327) -> (double precision float=w326:dbl)
            n104 = Subtract(x=w330, y=w329) -> (x-y=→"msec 1":u32)
          }
          frame #3 {
            # "Dev 2"
            n105 = case shown="\"Dev 2\", Default" w346 {
              tunnel: w349 -> [w365 _]
              tunnel: [w364 w440] -> w335
              tunnel: w348 -> [w363 _]
              tunnel: w347 -> [w362 w441]
              tunnel: w333 -> [w361 _]
              tunnel: w332 -> [w360 _]
              tunnel: w345 -> [w359 _]
              tunnel: [w358 w442] -> w331
              tunnel: [w357 w442] -> w334
              tunnel: [w356 w441] -> w342
              tunnel: [w355 w439] -> w343
              tunnel: w337 -> [w354 _]
              tunnel: [w353 w440] -> w336
              tunnel: w338 -> [w352 _]
              tunnel: w344 -> [w351 _]
              tunnel: w339 -> [w350 w439]
              frame "Dev 2", Default {
                n106 = case shown="False" w363 {
                  tunnel: w365 -> [w382 w424]
                  tunnel: [w380 w420] -> w355
                  tunnel: [w378 w431] -> w356
                  tunnel: w359 -> [w377 _]
                  tunnel: [w376 w430] -> w364
                  tunnel: [w375 w422] -> w357
                  tunnel: w362 -> [w369 w431]
                  tunnel: w354 -> [w370 w430]
                  tunnel: [w371 w428] -> w358
                  tunnel: w361 -> [w374 w427]
                  tunnel: w360 -> [w372 w426]
                  tunnel: [w368 w423] -> w353
                  tunnel: w352 -> [w367 w425]
                  tunnel: w351 -> [_ w421]
                  tunnel: w350 -> [w366 w420]
                  frame False {
                    n107 = case shown="True" w382 {
                      tunnel: w366 -> [w401 _]
                      tunnel: [w401 w417] -> w381
                      tunnel: [w402 w407] -> w379
                      tunnel: [w403 "Samps/Chl 2"] -> w376
                      tunnel: w370 -> [w403 _]
                      tunnel: w369 -> [w402 _]
                      tunnel: [w400 w408] -> w368
                      tunnel: w367 -> [w400 _]
                      frame False {
                      }
                      frame True {
                        # "Inits the A/D Task"
                        n108 = call <vilib>:"DAQmx Unflatten Channel String.vi"("names in"="PhyChls 2") -> ("names out"=w409:string[])  [unwired: 13 in, 1 out]
                        n109 = call-poly <vilib>:"DAQmx Create Virtual Channel.vi"("maximum value"="MaxVolts 2", "minimum value"="MiinVolts 2", "input terminal configuration"="InputCfg 2", "physical channels"="PhyChls 2", "error in"=errorcluster {"status"=FALSE, "code"=0, "source"=""}) -> ("task out"=w418:refnum<k21>, "error out"=w419:errorcluster)  [unwired: 9 in]
                        n110 = Array Size(array=w409) -> (size(s)=w408:i32)
                        "NumChls 3" <- w408
                        n111 = global write "Global ER2007.vi" "DAQ Init"(FALSE ("A/D Init")) -> ()
                        n112 = call-poly <vilib>:"DAQmx Timing.vi"("task/channels in"=w418, "sample mode"="SampleMode 2", "samples per channel"="Samps/Chl 2", "rate"="Rate 2", "error in"=w419) -> ("task out"=w407:refnum<k21>, "error out"=w417:errorcluster)  [unwired: 9 in]
                        n113 = property class="DAQmx Timing"(reference=w407) -> ("Sample Clock:Rate"=→"ActRate 2":dbl)  [unwired: 1 in, 2 out]
                      }
                    }
                    n114 = case shown="False" w377 {
                      tunnel: w381 -> [w391 w398]
                      tunnel: w379 -> [w390 w399]
                      tunnel: [w389 w399] -> w378
                      tunnel: [w387 w398] -> w380
                      tunnel: [w386 dbl[] [0.0, 0.0, 0.0, 0.0, 0.0, 0.0, 0.0, 0.0, 0.0, 0.0, 0.0, 0.0] ("data")] -> w375
                      tunnel: w376 -> [w384 _]
                      frame False {
                        n115 = call-poly <vilib>:"DAQmx Read.vi"("task/channels in"=w390, "number of samples per channel"=w384, "error in"=w391) -> ("task out"=w389:refnum<k21>, "data"=w385:dbl[][], "error out"=w388:errorcluster)  [unwired: 10 in]
                        n116 = for {
                          tunnel: [w396] -> w386 mode=indexing
                          tunnel: w385 -> [w395] mode=indexing
                          n117 = call-poly <vilib>:"Mean.vi"("X"=w395) -> ("mean"=w396:dbl)  [unwired: 1 out]
                        }
                        n118 = case shown="True" "T=Notify" {
                          tunnel: w388 -> [w392 w394]
                          tunnel: [w392 w393] -> w387
                          frame False {
                          }
                          frame True {
                            n119 = call <vilib>:"Simple Error Handler.vi"("error in (no error)"=w394) -> ("error out"=w393:errorcluster)  [unwired: 4 in, 4 out]
                          }
                        }
                      }
                      frame True {
                        # "Prev error"
                      }
                    }
                    n120 = Subtract(x=w375, y=w374) -> (x-y=w373:dbl[])
                    n121 = Multiply(x=w373, y=w372) -> (x*y=w371:dbl[])
                  }
                  frame True {
                    # "Dev 1 Assignments\n\nChl Desc  Dev Out Idx\n--------  -----------\n  NOP2          7\n  TC2A          8\n  TC2B          9\n  Pc2B         10\n  Pc3A         11\n  TC3A         12\n  TC3B         13\n  Pc2A         14\n  CJ2A         15\n  CJ2B         16\n  NOP3         17\n  Pc3B         18\n  CJ3A         19\n  CJ3B         20\n  NOP4         21\n  TC4A         22\n  TC4B         23\n  Pc4B         24\n  Pc5A         25\n  TC5A         26\n  TC5B         27\n  Pc4A         28\n  CJ4A         29\n  CJ4B         30\n  NOP5         31\n  Pc5B         32\n  CJ5A         33\n  CJ5B         34"
                    # "See templates\nto the left"
                    # "Sim for Dev 2"
                    n122 = case shown="True" w424 {
                      tunnel: w425 -> [w434 _]
                      tunnel: [w434 w436] -> w423
                      frame False {
                      }
                      frame True {
                        # "Init"
                        n123 = local read "PhyChls 2"() -> (w438:tag)
                        n124 = global write "Global ER2007.vi" "DAQ Init"(FALSE ("A/D Init")) -> ()
                        n125 = call <vilib>:"DAQmx Unflatten Channel String.vi"("names in"=w438) -> ("names out"=w437:string[])  [unwired: 13 in, 1 out]
                        n126 = Array Size(array=w437) -> (size(s)=w436:i32)
                        n127 = local write "NumChls 3"(w436) -> ()
                      }
                    }
                    n128 = case shown="Default" w421 {
                      tunnel: [w432 w433] -> w422
                      frame "Cell 2" {
                        w432 = dbl[] [2.2, 0.42, 0.43, 1.89, 0.002, 0.001, 0.004, 3.45, 1.25, 1.25, -0.004, -0.003, 0.003, 0.002, -0.005, 0.003, 0.007, -0.004, 0.002, 0.002, 0.004, 0.0, 1.25, 1.25, -0.005, 0.005, 1.25, 1.25]  # Cell 2 Active
                      }
                      frame Default {
                        w433 = dbl[] [0.001, -0.001, -0.001, -0.002, -0.001, -0.001, 0.002, 0.011, 1.25, 1.25, 0.003, 1.25, 1.25, 0.001, 0.004, 0.005, 0.009, 0.005, 0.006, 0.007, 0.007, 0.008, 1.25, 1.25, 0.008, 1.25, 1.25, 0.009, 1.25, 1.25]  # None Active
                      }
                    }
                    n129 = Subtract(x=w422, y=w427) -> (x-y=w429:dbl[])
                    n130 = Multiply(x=w429, y=w426) -> (x*y=w428:dbl[])
                  }
                }
              }
              frame "Dev 1", "Galil" {
                w442 = dbl[] []
                w440 = 0 ("Samps/Chl")
              }
            }
            n131 = Not(x=w341) -> (.not. x?=w340:bool)
            "Sample 2" <- w340
          }
          frame #4 {
            n132 = Tick Count (ms)() -> (millisecond timer value=w444:u32)
            n133 = Subtract(x=w444, y=w445) -> (x-y=→"msec 2":u32)
          }
          frame #5 {
            # "Galil"
            n134 = case shown="\"Galil\", Default" w457 {
              tunnel: w465 -> [_ w490]
              tunnel: w464 -> [_ w489]
              tunnel: w463 -> [_ w488]
              tunnel: w462 -> [_ w487]
              tunnel: [w471 w486] -> w450
              tunnel: [w471 w485] -> w451
              tunnel: [0 ("Samps/Chl") w484] -> w461
              tunnel: w460 -> [w469 w483]
              tunnel: [w469 w482] -> w446
              tunnel: w459 -> [w470 w481]
              tunnel: [w470 w480] -> w458
              tunnel: [u16[] [1, 2, 3, 4, 5] ("Controller #'s") w479] -> w456
              tunnel: w455 -> [_ w478]
              tunnel: w454 -> [_ w477]
              tunnel: w453 -> [_ w476]
              tunnel: w452 -> [w467 w475]
              tunnel: [w467 w474] -> w449
              tunnel: w448 -> [_ w473]
              tunnel: w447 -> [_ w472]
              frame "Dev 1".."Dev 1 & Dev 2" {
                w471 = dbl[] []
                # "Galil not active"
              }
              frame "Galil", Default {
                n135 = stacked-sequence {
                  seq-local: [w492 _] -> [_ w516]
                  tunnel: w490 -> [w496 w531]
                  tunnel: w489 -> [_ w530]
                  tunnel: w488 -> [_ w529]
                  tunnel: w487 -> [_ w528]
                  tunnel: [_ w527] -> w486
                  tunnel: [_ w526] -> w485
                  tunnel: [_ w525] -> w484
                  tunnel: w483 -> [_ w524]
                  tunnel: [_ w523] -> w482
                  tunnel: w481 -> [_ w522]
                  tunnel: [_ w521] -> w480
                  tunnel: [_ w520] -> w479
                  tunnel: w478 -> [_ w519]
                  tunnel: w477 -> [_ w518]
                  tunnel: w476 -> [_ w517]
                  tunnel: w475 -> [w495 _]
                  tunnel: [w493 _] -> w474
                  tunnel: w473 -> [w494 _]
                  tunnel: w472 -> [w491 w515]
                  frame #0 {
                    # "next time"
                    # "current time"
                    # "Galil interval timing"
                    n136 = case shown="False" w496 {
                      tunnel: "Period 3" -> [w503 w512]
                      tunnel: w495 -> [w502 _]
                      tunnel: w494 -> [w501 w513]
                      tunnel: [w500 w514] -> w493
                      tunnel: [w499 w511] -> w492
                      tunnel: w491 -> [w498 _]
                      frame False {
                        n137 = Greater Or Equal?(x=w501, y=w502) -> (x >= y?=w504:bool)
                        n138 = case shown="True" w504 {
                          tunnel: w501 -> [_ w508]
                          tunnel: [w505 w510] -> w499
                          tunnel: [w506 w509] -> w500
                          tunnel: w502 -> [w506 _]
                          tunnel: w503 -> [_ w507]
                          tunnel: w498 -> [w505 _]
                          frame False {
                            # "not time yet"
                          }
                          frame True {
                            w510 = TRUE  # Query now
                            n139 = Add(x=w508, y=w507) -> (x+y=w509:dbl)
                          }
                        }
                      }
                      frame True {
                        w511 = TRUE  # Query now
                        # "Initialization"
                        n140 = Add(x=w513, y=w512) -> (x+y=w514:dbl)
                      }
                    }
                    "Query" <- w492
                  }
                  frame #1 {
                    n141 = case shown="True" w517 {
                      tunnel: w531 -> [w552 w661]
                      tunnel: [w550 w653] -> w523
                      tunnel: [w539 w665] -> w521
                      tunnel: w524 -> [w549 w654]
                      tunnel: [w543 w664] -> w525
                      tunnel: w522 -> [w539 w665]
                      tunnel: w530 -> [w547 w664]
                      tunnel: [w546 w662] -> w527
                      tunnel: w529 -> [w540 w655]
                      tunnel: w528 -> [w541 w656]
                      tunnel: [w545 w658] -> w526
                      tunnel: [w542 w659] -> w520
                      tunnel: w519 -> [w544 w660]
                      tunnel: w518 -> [_ w657]
                      tunnel: w516 -> [w536 _]
                      tunnel: w515 -> [w537 _]
                      frame False {
                        n142 = case shown="True" w552 {
                          tunnel: w549 -> [w642 _]
                          tunnel: [w642 errorcluster {"status"=FALSE, "code"=0, "source"=""} ("error out")] -> w551
                          tunnel: [w644 w648] -> w543
                          tunnel: w547 -> [w644 _]
                          tunnel: [w643 "Controller #'s"] -> w542
                          tunnel: w544 -> [w643 _]
                          tunnel: [w641 w647] -> w538
                          tunnel: [FALSE ("status") FALSE ("status")] -> w532
                          frame False {
                            w641 = FALSE  # Init
                          }
                          frame True {
                            w647 = TRUE  # Init
                            # "Init"
                            # "Inits the A/D Task"
                            n143 = Array Size(array="Controller #'s") -> (size(s)=w648:i32)
                            "NumCtrls" <- w648
                            n144 = global write "Global ER2007.vi" "DAQ Init"(FALSE ("A/D Init")) -> ()
                            n145 = Multiply(x=2, y=w648) -> (x*y=→"NumChls 3":i32)
                          }
                        }
                        n146 = global read "Global ER2007.vi" "No Galil"() -> (w535:bool[])
                        n147 = Array Subset(array=w535, index=1) -> (w533:bool[])  [unwired: 1 in]
                        n148 = case shown="True" w536 {
                          tunnel: w551 -> [w553 w563]
                          tunnel: [w553 w562] -> w550
                          tunnel: w532 -> [_ w561]
                          tunnel: [w554 w560] -> w545
                          tunnel: w543 -> [_ w559]
                          tunnel: w542 -> [_ w558]
                          tunnel: w533 -> [_ w555]
                          tunnel: w538 -> [_ w557]
                          tunnel: w537 -> [_ w556]
                          frame False {
                            # "Not time to sample"
                            n149 = local read "EUs 3"() -> (w554:dbl[])
                          }
                          frame True {
                            # "Time to sample"
                            n150 = case shown="False" w561 {
                              tunnel: w563 -> [w570 w639]
                              tunnel: [w574 w639] -> w562
                              tunnel: [w567 dbl[] [0.0, 0.0, 0.0, 0.0, 0.0, 0.0, 0.0, 0.0, 0.0, 0.0, 0.0, 0.0] ("data")] -> w560
                              tunnel: w559 -> [w572 _]
                              tunnel: w558 -> [w571 _]
                              tunnel: w557 -> [w566 _]
                              tunnel: w556 -> [w565 _]
                              tunnel: w555 -> [w564 _]
                              frame False {
                                n151 = for {
                                N: w572 -> [_]
                                tunnel: w571 -> [w579] mode=indexing
                                shift-right: [w586] -> w569
                                shift-left: w570 -> [w587]
                                shift-right: [w581] -> w567
                                shift-left: dbl[] [] -> [w583]
                                tunnel: w566 -> [w578]
                                tunnel: w565 -> [w577]
                                tunnel: w564 -> [w576] mode=indexing
                                i -> [w575]
                                n152 = case shown="1" w579 {
                                selector: w579 -> [_ w594 w606 w615 w624 w631]
                                tunnel: w587 -> [w589 w598 w601 w614 w623 w633]
                                tunnel: [w589 w597 w603 w613 w622 w632] -> w586
                                tunnel: [w588 w596 w607 w616 w625 w634] -> w585
                                tunnel: [w588 w595 w602 w612 w621 w630] -> w584
                                tunnel: w578 -> [_ w593 w605 w611 w620 w629]
                                tunnel: w577 -> [_ w592 w604 w610 w619 w628]
                                tunnel: w576 -> [_ w591 w600 w609 w618 w627]
                                tunnel: w575 -> [_ w590 w599 w608 w617 w626]
                                frame 0, Default {
                                w588 = 0.0 ("Delta-P")
                                }
                                frame 1 {
                                n153 = call "Get VPA 1 Values.vi"("Controller #"=w594, "No Galil"=w591, "ErrIn"=w598, "Iteration"=w590, "Initialize"=w593, "Stop"=w592) -> ("Delta-P"=w596:dbl, "Volume"=w595:dbl, "ErrOut"=w597:errorcluster)  [unwired: 6 in, 1 out]
                                }
                                frame 2 {
                                n154 = call "Get VPA 2 Values.vi"("Controller #"=w606, "No Galil"=w600, "ErrIn"=w601, "Iteration"=w599, "Initialize"=w605, "Stop"=w604) -> ("Delta-P"=w607:dbl, "Volume"=w602:dbl, "ErrOut"=w603:errorcluster)  [unwired: 6 in, 1 out]
                                }
                                frame 3 {
                                n155 = call "Get VPA 3 Values.vi"("Controller #"=w615, "No Galil"=w609, "ErrIn"=w614, "Iteration"=w608, "Initialize"=w611, "Stop"=w610) -> ("Delta-P"=w616:dbl, "Volume"=w612:dbl, "ErrOut"=w613:errorcluster)  [unwired: 6 in, 1 out]
                                }
                                frame 4 {
                                n156 = call "Get VPA 4 Values.vi"("Controller #"=w624, "No Galil"=w618, "ErrIn"=w623, "Iteration"=w617, "Initialize"=w620, "Stop"=w619) -> ("Delta-P"=w625:dbl, "Volume"=w621:dbl, "ErrOut"=w622:errorcluster)  [unwired: 6 in, 1 out]
                                }
                                frame 5 {
                                n157 = call "Get VPA 5 Values.vi"("Controller #"=w631, "No Galil"=w627, "ErrIn"=w633, "Iteration"=w626, "Initialize"=w629, "Stop"=w628) -> ("Delta-P"=w634:dbl, "Volume"=w630:dbl, "ErrOut"=w632:errorcluster)  [unwired: 6 in, 1 out]
                                }
                                }
                                n158 = Build Array(w585, w584) -> (w582:dbl[])
                                n159 = Build Array (concatenate)(w583, w582) -> (w581:dbl[])
                                n160 = Wait (ms)(milliseconds to wait=u32 20) -> ()  [unwired: 1 out]
                                }
                                n161 = case shown="True" "T= Log Error" {
                                tunnel: w569 -> [w635 w637]
                                tunnel: [w635 w636] -> w574
                                frame False {
                                }
                                frame True {
                                n162 = call "Write VPA Error Log File.vi"("Error In"=w637) -> ("Error Out"=w636:errorcluster)  [unwired: 7 in, 3 out]
                                }
                                }
                              }
                              frame True {
                                # "Error"
                              }
                            }
                          }
                        }
                        n163 = Divide(x=w545, y=w541) -> (x/y=w548:dbl[])
                        n164 = Add(x=w548, y=w540) -> (x+y=w546:dbl[])
                      }
                      frame True {
                        # "Galil Assignments\n\nChl Desc  Dev Out Idx  Both Out Idx\n--------  -----------  ------------\n  Pdp1          0           30\n Pvol1          1           31\n  Pdp2          2           32\n Pvol2          3           33\n  Pdp3          4           34\n Pvol3          5           35\n  Pdp4          6           36\n Pvol4          7           37\n  Pdp5          8           38\n Pvol5          9           39"
                        # "Sim Galil"
                        n165 = case shown="True" w661 {
                          tunnel: w660 -> [w669 _]
                          tunnel: [w669 u16[] [1, 2, 3, 4, 5] ("Controller #'s")] -> w659
                          tunnel: w654 -> [w668 _]
                          tunnel: [w668 errorcluster {"status"=FALSE, "code"=0, "source"=""} ("error out")] -> w653
                          frame False {
                          }
                          frame True {
                            # "Init"
                            n166 = local write "NumChls 3"(10 ("NumChls 2")) -> ()
                            n167 = global write "Global ER2007.vi" "DAQ Init"(FALSE ("A/D Init")) -> ()
                          }
                        }
                        n168 = case shown="\"Cell 2\"" w657 {
                          tunnel: [w666 w667] -> w658
                          frame Default {
                            w666 = dbl[] [0.001, -0.001, 0.002, -0.002, 0.003, -0.003, 0.004, -0.004, 0.005, -0.005]  # None Active
                          }
                          frame "Cell 2" {
                            w667 = dbl[] [0.001, -0.001, 222.0, 11.0, 0.003, -0.003, 0.004, -0.004, 0.005, -0.005]  # Cell Active
                          }
                        }
                        n169 = Divide(x=w658, y=w656) -> (x/y=w663:dbl[])
                        n170 = Add(x=w663, y=w655) -> (x+y=w662:dbl[])
                      }
                    }
                  }
                }
              }
            }
          }
          frame #6 {
            n171 = Tick Count (ms)() -> (millisecond timer value=w676:u32)
            n172 = Subtract(x=w676, y=w674) -> (x-y=→"msec 3":u32)
          }
          frame #7 {
            # "EUs 2"
            # "Volts 2"
            # "Dev2 Error"
            # "Volts 3"
            # "EUs 3"
            # "Volts 1"
            # "EUs 1"
            # "Final values"
            n173 = Index Array(array="TC & CJ-1 Idxs", index (col) #1=0 ("disabled index (col)")) -> (element #1=w700:i32[], element #2=w699:i32[])  [unwired: 3 in]
            n174 = global write "Global ER2007.vi" "DAQ Run"(TRUE ("A/D Run")) -> ()
            n175 = case shown="No Error" w683 {
              selector: w683 -> [_ w724]
              tunnel: w691 -> [w717 w725]
              tunnel: [w714 w725] -> w690
              tunnel: [w716 w724] -> w692
              tunnel: w682 -> [w715 _]
              frame No Error {
                n176 = case shown="No Error" w715 {
                  selector: w715 -> [_ w723]
                  tunnel: w717 -> [w718 w722]
                  tunnel: [w719 w723] -> w716
                  tunnel: [w718 w722] -> w714
                  frame No Error {
                    n177 = case shown="No Error" w718 {
                      selector: w718 -> [w720 w721]
                      tunnel: [w720 w721] -> w719
                      frame No Error {
                      }
                      frame Error {
                      }
                    }
                  }
                  frame Error {
                  }
                }
              }
              frame Error {
              }
            }
            "ErrOut" <- w692
            n178 = Unbundle By Name(w683) -> ("status"=w680:bool)
            "Dev1 Err" <- w680
            n179 = Unbundle By Name(w682) -> ("status"=w681:bool)
            "Dev2 Err" <- w681
            n180 = Or(x=w680, y=w681) -> (x .or. y?=w679:bool)
            n181 = Build Array (concatenate)(w685, w678) -> (w686:dbl[])
            n182 = for {
              tunnel: w700 -> [w706] mode=indexing
              shift-right: [w709] -> w698
              shift-left: w686 -> [w711]
              tunnel: w699 -> [w705] mode=indexing
              tunnel: "ThermocoupleType" -> [w704]
              n183 = Index Array(array=w711, index #1=w706, index #2=w705) -> (element #1=w713:dbl, element #2=w712:dbl)
              n184 = call "SCC-TC0x Calculate Temperatures.vi"("ThermocoupleType"=w704, "CJC Voltage"=w712, "T/C Voltage"=w713) -> ("CJ Temperature"=w707:dbl, "T/C Temperature"=w708:dbl)  [unwired: 6 in, 1 out]
              n185 = Replace Array Subset(array=w711, new element=w708, index=w706) -> (w710:dbl[])
              n186 = Replace Array Subset(array=w710, new element=w707, index=w705) -> (w709:dbl[])
            }
            n187 = Build Array (concatenate)(w698, w684) -> (w694:dbl[])
            n188 = global write "Global ER2007.vi" "A/D EUs"(w694) -> ()
            n189 = global write "Global ER2007.vi" "A/D Err"(w679) -> ()
            n190 = Unbundle By Name(w691) -> ("status"=w689:bool)
            "Galil Err" <- w689
            n191 = Build Array (concatenate)(w703, w687, w688) -> (w695:dbl[])
            n192 = global write "Global ER2007.vi" "A/D Volts"(w695) -> ()
            n193 = global write "Global ER2007.vi" "Galil Err"(w689) -> ()
            "Volts 1" <- w703
            "Late" <- w702
            "EUs 3" <- w684
            "EUs 1" <- w685
            "EUs 2" <- w678
            "Volts 2" <- w687
          }
          frame #8 {
            # "Checks if \"NewCals\" and updates shift registers if TRUE"
            n194 = global read "Global ER2007.vi" "NewCals"() -> (w738:bool)
            n195 = case shown="True" w738 {
              tunnel: w737 -> [w744 _]
              tunnel: w736 -> [w742 _]
              tunnel: [w744 w750] -> w735
              tunnel: w734 -> [w743 _]
              tunnel: [w743 w745] -> w727
              tunnel: [w742 w749] -> w728
              tunnel: w733 -> [w741 _]
              tunnel: [w741 w746] -> w732
              tunnel: w731 -> [w740 _]
              tunnel: [w740 w747] -> w726
              tunnel: w730 -> [w739 _]
              tunnel: [w739 w748] -> w729
              frame False {
              }
              frame True {
                n196 = stacked-sequence {
                  seq-local: [w755 _] -> [_ w840]
                  tunnel: [_ w839] -> w750
                  tunnel: [_ w838] -> w749
                  tunnel: [w754 _] -> w748
                  tunnel: [w753 _] -> w747
                  tunnel: [w752 _] -> w746
                  tunnel: [w751 _] -> w745
                  frame #0 {
                    w760 = "<spare>" ("x")
                    # "A/D Cal K's"
                    # "PCI-6220 A/D chls 0:15"
                    # "PCI-6224 A/D chls 16:32"
                    # "PCI-6224 A/D chls 0:15"
                    n197 = global read "Global ER2007.vi" "CalData"() -> (w755:T5)
                    n198 = global read "Global ER2007.vi" "A/D Pages"() -> (w769:i32[])
                    n199 = Index Array(array=w769, index #1=0 ("index")) -> (element #1=w758:i32, element #2=w756:i32, element #3=w757:i32)  [unwired: 2 in]
                    n200 = Index Array(array=w755, index=w758) -> (element=w764:T6)
                    n201 = Index Array(array=w755, index=w756) -> (element=w777:T6)
                    n202 = Index Array(array=w755, index=w757) -> (element=w779:T6)
                    n203 = Unbundle By Name(w764) -> ("ChlDesc"=w763:string[], "ChlZero"=w762:sgl[], "ChlFactor"=w761:sgl[])
                    n204 = Unbundle By Name(w777) -> ("ChlDesc"=w776:string[], "ChlZero"=w775:sgl[], "ChlFactor"=w774:sgl[])
                    n205 = Unbundle By Name(w779) -> ("ChlDesc"=w770:string[], "ChlZero"=w771:sgl[], "ChlFactor"=w772:sgl[])
                    n206 = Initialize Array(0.0 ("element")) -> (w759:dbl[])  [unwired: 1 in]
                    n207 = for {
                      tunnel: w763 -> [w790] mode=indexing
                      tunnel: w762 -> [w783] mode=indexing
                      tunnel: w761 -> [w782] mode=indexing
                      tunnel: w760 -> [w789]
                      shift-right: [w786] -> w753
                      shift-left: w759 -> [w787]
                      shift-right: [w784] -> w754
                      shift-left: w759 -> [w785]
                      n208 = To Double Precision Float(number=w783) -> (double precision float=w781:dbl)
                      n209 = To Double Precision Float(number=w782) -> (double precision float=w780:dbl)
                      n210 = Equal?(x=w789, y=w790) -> (x = y?=w788:bool)
                      n211 = case shown="False" w788 {
                        tunnel: w787 -> [w796 w798]
                        tunnel: [w794 w798] -> w786
                        tunnel: w785 -> [w792 w797]
                        tunnel: [w793 w797] -> w784
                        tunnel: w781 -> [w795 _]
                        tunnel: w780 -> [w791 _]
                        frame False {
                          n212 = Build Array (concatenate)(w796, w795) -> (w794:dbl[])
                          n213 = Build Array (concatenate)(w792, w791) -> (w793:dbl[])
                        }
                        frame True {
                          # "<spare> chl"
                        }
                      }
                    }
                    n214 = for {
                      tunnel: w776 -> [w828] mode=indexing
                      tunnel: w775 -> [w821] mode=indexing
                      tunnel: w774 -> [w820] mode=indexing
                      tunnel: w760 -> [w827]
                      shift-right: [w824] -> w767
                      shift-left: w759 -> [w825]
                      shift-right: [w822] -> w765
                      shift-left: w759 -> [w823]
                      n215 = To Double Precision Float(number=w821) -> (double precision float=w819:dbl)
                      n216 = To Double Precision Float(number=w820) -> (double precision float=w818:dbl)
                      n217 = Equal?(x=w827, y=w828) -> (x = y?=w826:bool)
                      n218 = case shown="True" w826 {
                        tunnel: w825 -> [w834 w836]
                        tunnel: [w832 w836] -> w824
                        tunnel: w823 -> [w830 w835]
                        tunnel: [w831 w835] -> w822
                        tunnel: w819 -> [w833 _]
                        tunnel: w818 -> [w829 _]
                        frame False {
                          n219 = Build Array (concatenate)(w834, w833) -> (w832:dbl[])
                          n220 = Build Array (concatenate)(w830, w829) -> (w831:dbl[])
                        }
                        frame True {
                          # "<spare> chl"
                        }
                      }
                    }
                    n221 = for {
                      tunnel: w770 -> [w809] mode=indexing
                      tunnel: w771 -> [w802] mode=indexing
                      tunnel: w772 -> [w801] mode=indexing
                      tunnel: w760 -> [w808]
                      shift-right: [w805] -> w768
                      shift-left: w759 -> [w806]
                      shift-right: [w803] -> w766
                      shift-left: w759 -> [w804]
                      n222 = To Double Precision Float(number=w802) -> (double precision float=w800:dbl)
                      n223 = To Double Precision Float(number=w801) -> (double precision float=w799:dbl)
                      n224 = Equal?(x=w808, y=w809) -> (x = y?=w807:bool)
                      n225 = case shown="False" w807 {
                        tunnel: w806 -> [w815 w817]
                        tunnel: [w813 w817] -> w805
                        tunnel: w804 -> [w811 w816]
                        tunnel: [w812 w816] -> w803
                        tunnel: w800 -> [w814 _]
                        tunnel: w799 -> [w810 _]
                        frame False {
                          n226 = Build Array (concatenate)(w815, w814) -> (w813:dbl[])
                          n227 = Build Array (concatenate)(w811, w810) -> (w812:dbl[])
                        }
                        frame True {
                          # "<spare> chl"
                        }
                      }
                    }
                    n228 = Build Array (concatenate)(w767, w768) -> (w751:dbl[])
                    n229 = Build Array (concatenate)(w765, w766) -> (w752:dbl[])
                  }
                  frame #1 {
                    # "Galil Cal K's"
                    n230 = global read "Global ER2007.vi" "Galil Pages"() -> (w845:i32[])
                    n231 = Index Array(array=w845, index=0) -> (element=w847:i32)
                    n232 = Index Array(array=w840, index=w847) -> (element=w841:T6)
                    n233 = Unbundle By Name(w841) -> ("ChlDesc"=w842:string[], "ChlZero"=w843:sgl[], "ChlFactor"=w844:sgl[])
                    n234 = Initialize Array(0.0 ("element")) -> (w850:dbl[])  [unwired: 1 in]
                    n235 = global write "Global ER2007.vi" "NewCals"(FALSE ("NewCals")) -> ()
                    n236 = for {
                      tunnel: w842 -> [w861] mode=indexing
                      tunnel: w843 -> [w854] mode=indexing
                      tunnel: w844 -> [w853] mode=indexing
                      tunnel: "<spare>" ("x") -> [w860]
                      shift-right: [w857] -> w839
                      shift-left: w850 -> [w858]
                      shift-right: [w855] -> w838
                      shift-left: w850 -> [w856]
                      n237 = To Double Precision Float(number=w854) -> (double precision float=w852:dbl)
                      n238 = To Double Precision Float(number=w853) -> (double precision float=w851:dbl)
                      n239 = Equal?(x=w860, y=w861) -> (x = y?=w859:bool)
                      n240 = case shown="False" w859 {
                        tunnel: w858 -> [w867 w869]
                        tunnel: [w865 w869] -> w857
                        tunnel: w856 -> [w863 w868]
                        tunnel: [w864 w868] -> w855
                        tunnel: w852 -> [w866 _]
                        tunnel: w851 -> [w862 _]
                        frame False {
                          n241 = Build Array (concatenate)(w867, w866) -> (w865:dbl[])
                          n242 = Build Array (concatenate)(w863, w862) -> (w864:dbl[])
                        }
                        frame True {
                          # "<spare> chl"
                        }
                      }
                    }
                  }
                }
              }
            }
          }
        }
      }
      n243 = node-c288(w134) -> ()  [unwired: 1 out]
    }
    frame #2 {
      w874 = FALSE ("A/D Stop")
      # "Clears the A/D task and globals"
      n244 = global write "Global ER2007.vi" "DAQ Stop"(w874) -> ()
      n245 = global write "Global ER2007.vi" "DAQ Run"(w874) -> ()
      n246 = call <vilib>:"DAQmx Clear Task.vi"("task in"=w875) -> ()  [unwired: 14 in, 1 out]
      n247 = call <vilib>:"DAQmx Clear Task.vi"("task in"=w876) -> ()  [unwired: 14 in, 1 out]
      n248 = call <vilib>:"DAQmx Clear Task.vi"("task in"=w873) -> ()  [unwired: 14 in, 1 out]
    }
  }
